vi "DtCreateCtrOneShotChan.vi"(1 "Requested\nPulse Width  (msecs)":dbl=1.0, 2 "Pulse Polarity":i32(ring)=601 items=["HighToLow"=600, "LowToHigh"=601], 5 "Board Name":string, 7 "Counter Num":u32, 9 "Trigger":i32(ring) items=["RisingEdge", "FallingEdge", "Immediate"], 11 "error in (no error)":errorcluster) -> (4 "Task out":i32, 6 "Actual Pulse \nWidth  (msecs)":dbl, 15 "error out":errorcluster)   [LabVIEW 2016]
doc: "Creates one or more virtual counter/timer channels that output a single pulse for a specified duration (in milliseconds) the first time that the device detects a trigger (determined by the counter/timer's gate input signal). You can use this pulse output signal as an external digital (TTL) trigger for other tasks, such as analog input or analog output tasks. This type of task is also known as a one-shot.\n\nOnce you have created a virtual counter/timer channel for a one-shot task, use the DtOLStart VI to start the task. To output another value, use the DtOLReStart VI to restart the task.\n\nWhen the counter/timer is triggered, a single pulse is output; then, the one-shot task stops. All subsequent gate input signals to the counter/timer are ignored."
uses:
  <userlib>/LV-Link3/DtLvLink.lvlib
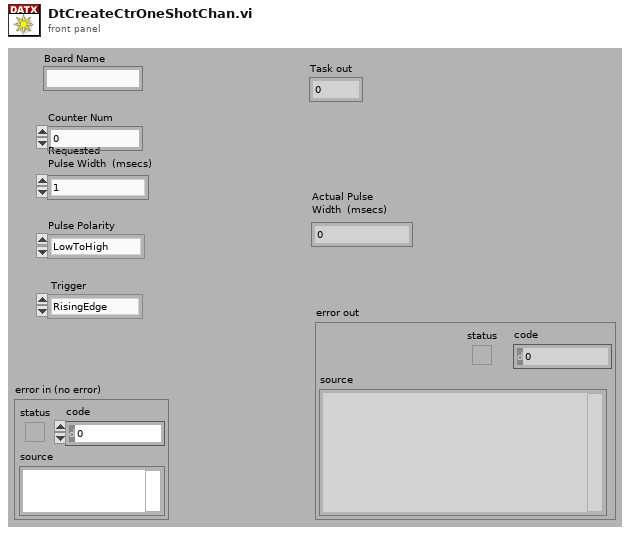
[diagram p1: front panel]
types:
  T1 = enum32{"AnalogInput", "AnalogOutput", "DigitalInput", "DigitalOutput", "Quadrature", "CounterTimer"}
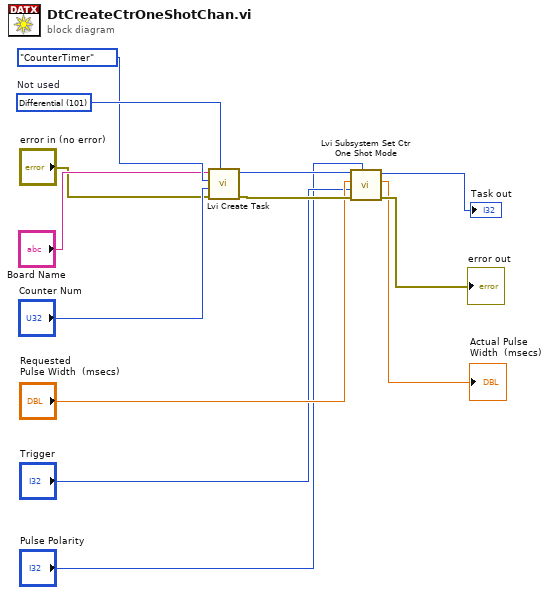
[diagram p0: block diagram]
diagram:
  w13 = 101 items=["SingleEnded"=100, "Differential"=101]  # Not used
  n1 = call <userlib>:"Lvi Create Task.vi"("SEorDiff"=w13, "error in (no error)"="error in (no error)", "SubSysIndex"="Counter Num", "ChanType"=T1."CounterTimer", "BoardName"="Board Name") -> ("error out"=w7:errorcluster, "TaskRef"=w6:i32)  [unwired: 4 in, 1 out]
  n2 = call <userlib>:"Lvi Subsystem Set Ctr One Shot Mode.vi"("Polarity"="Pulse Polarity", "error in (no error)"=w7, "CurGateType"="Trigger", "Millisecs"="Requested\nPulse Width  (msecs)", "TaskRef"=w6) -> ("error out"=→"error out":errorcluster, "ActualMillisecs"=→"Actual Pulse \nWidth  (msecs)":dbl, "TaskRef out"=→"Task out":i32)  [unwired: 3 in, 1 out]
